vi "From Config.vi"(5 "Copy Data? [T]":bool=TRUE, 7 "Copy Paths? [T]":bool=TRUE, 8 "error in (no error)":errorcluster, 10 "Carya Config src":refnum<class "Carya Config.lvclass">, 11 "Carya Config dst":refnum<class "Carya Config.lvclass">) -> (0 "error out":errorcluster, 2 "Carya Config src":refnum<class "Carya Config.lvclass">, 3 "Carya Config dst":refnum<class "Carya Config.lvclass">)   [LabVIEW 2013, in "Carya Config.lvclass"]
doc: "Copyright 2018, Carya Automatisering, Wiebe Walstra."
uses:
  Carya Config.lvclass
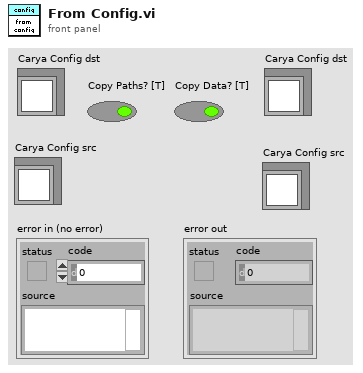
[diagram p1: front panel]
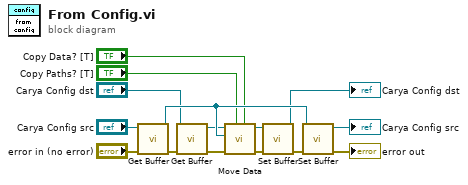
[diagram p0: block diagram]
diagram:
  n1 = call-dynamic "Get Buffer.vi"("error in (no error)"="error in (no error)", "Carya Config in"="Carya Config src") -> ("error out"=w4:errorcluster, "Config"=w11:refnum<class "Carya Config.lvclass">)  [unwired: 8 in]
  n2 = call-dynamic "Get Buffer.vi"("error in (no error)"=w4, "Carya Config in"="Carya Config dst") -> ("error out"=w7:errorcluster, "Config"=w10:refnum<class "Carya Config.lvclass">)  [unwired: 8 in]
  n3 = call "Move Data.vi"("Copy Data? [T]"="Copy Data? [T]", "Copy Paths? [T]"="Copy Paths? [T]", "error in (no error)"=w7, "Carya Config source"=w11, "Carya Config dest"=w10) -> ("error out"=w8:errorcluster, "Carya Config out"=w9:refnum<class "Carya Config.lvclass">)  [unwired: 5 in]
  n4 = call-dynamic "Set Buffer.vi"("error in (no error)"=w8, "Carya Config"=w9) -> ("error out"=w3:errorcluster, "Carya Config out"=→"Carya Config dst":refnum<class "Carya Config.lvclass">)  [unwired: 8 in]
  n5 = call-dynamic "Set Buffer.vi"("error in (no error)"=w3, "Carya Config"=w11) -> ("error out"=→"error out":errorcluster, "Carya Config out"=→"Carya Config src":refnum<class "Carya Config.lvclass">)  [unwired: 8 in]
